vi "Update Chart.vi"(8 "error in (no error)":errorcluster, 10 "Variant":variant, 11 "MultiSubscriber in":refnum<class "MultiSubscriber.lvclass">) -> (0 "error out":errorcluster, 3 "MultiSubscriber out":refnum<class "MultiSubscriber.lvclass">)   [LabVIEW 2018, in "TestViewables.lvlib" / "MultiSubscriber.lvclass"]
doc: "<License>\nCopyright © 2017 Composed Systems, LLC | All rights reserved\nwww.composed.io\n\nAuthor: Ethan Stern <ethan.stern@composed.io>\n\nThis software is provided \"AS IS\" WITHOUT WARRANTIES, either express or implied, AND IS FOR EDUCATIONAL PURPOSES ONLY.\n</License>"
uses:
  MultiSubscriber.lvclass
  modules/mva-viewable/Source/IViewable/IViewable/IViewable.lvclass
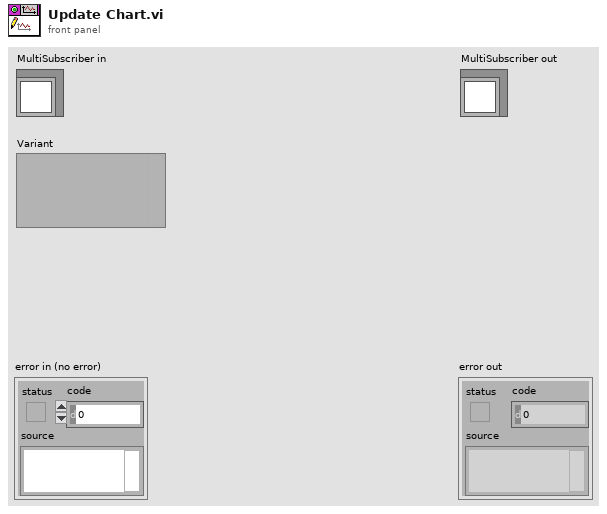
[diagram p1: front panel]
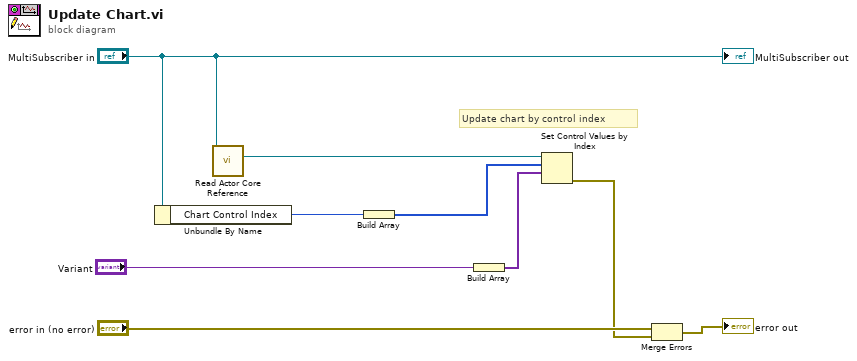
[diagram p0: block diagram]
diagram:
  # "Update chart by control index"
  n1 = Unbundle By Name("MultiSubscriber in") -> ("Chart Control Index"=w4:i32)
  n2 = call "Read Actor Core Reference.vi"("IViewable In"="MultiSubscriber in") -> ("Actor Core Refnum"=w7:refnum<vi>)  [unwired: 9 in, 1 out]
  n3 = Build Array(w4) -> (w3:i32[])
  n4 = Build Array("Variant") -> (w5:variant[])
  n5 = Set Control Values by Index(0:w7, 1:w3, 2:w5) -> (11:w2:errorcluster)  [unwired: 1 in]
  n6 = Merge Errors("error in (no error)", w2) -> (→"error out":errorcluster)
  "MultiSubscriber out" <- "MultiSubscriber in"
